vi "HelloWorld.vi"() -> ()   [LabVIEW 2024]
panel:
  out "str":string
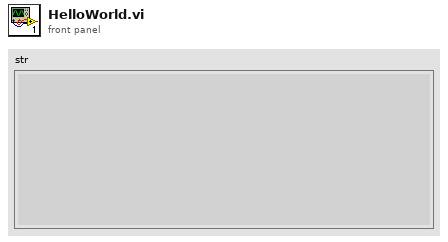
[diagram p1: front panel]
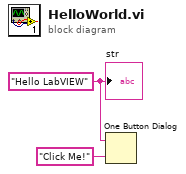
[diagram p0: block diagram]
diagram:
  w1 = "Hello LabVIEW"
  n1 = One Button Dialog(message=w1, button name ("OK")="Click Me!" ("String")) -> ()  [unwired: 1 out]
  "str" <- w1
